vi "Generate Fully Qualified Channel Names.vi"() -> (1 "Rx channels":string[](array[string]), 2 "trigger channels":string[](array[string]), 3 "Tx channels":string[](array[string]), 4 "channel index":dbl[](array[numeric]))   [LabVIEW 2020, in "Single Core Acyclic Loopback.lvclass"]
uses:
  Single Core Acyclic Loopback.lvclass
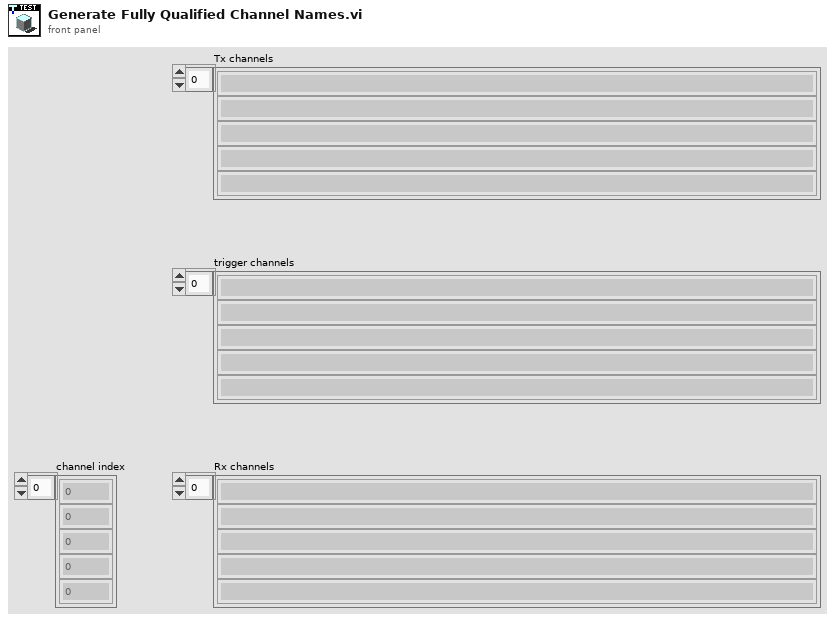
[diagram p1: front panel]
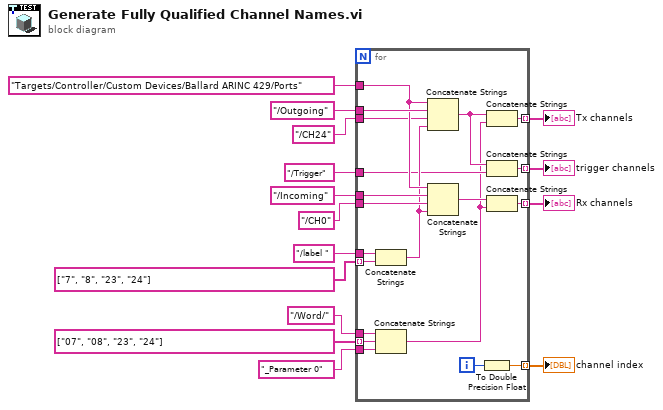
[diagram p0: block diagram]
diagram:
  n1 = for {
    tunnel: [w35] -> w14 mode=indexing
    tunnel: "Targets/Controller/Custom Devices/Ballard ARINC 429/Ports" ("Channel") -> [w27]
    tunnel: string[] ["07", "08", "23", "24"] -> [w33] mode=indexing
    tunnel: "_Parameter 0" ("format string") -> [w32]
    tunnel: "/label " ("format string") -> [w31]
    tunnel: string[] ["7", "8", "23", "24"] -> [w30] mode=indexing
    tunnel: "/Word/" ("input 1") -> [w29]
    tunnel: "/Outgoing" ("format string") -> [w28]
    tunnel: "/Incoming" ("format string") -> [w26]
    tunnel: "/CH0" ("format string") -> [w25]
    tunnel: "/CH24" ("format string") -> [w24]
    tunnel: "/Trigger" ("input 1") -> [w22]
    tunnel: [w21] -> w3 mode=indexing
    tunnel: [w17] -> w2 mode=indexing
    tunnel: [w16] -> w1 mode=indexing
    i -> [w34]
    n2 = Concatenate Strings(w31, w30) -> (w23:string)
    n3 = Concatenate Strings(w29, w33, w32) -> (w18:string)
    n4 = Concatenate Strings(w27, w28, w24, w23) -> (w19:string)
    n5 = Concatenate Strings(w27, w26, w25, w23) -> (w20:string)
    n6 = To Double Precision Float(number=w34) -> (double precision float=w35:dbl)
    n7 = Concatenate Strings(w19, w18) -> (w16:string)
    n8 = Concatenate Strings(w19, w22) -> (w21:string)
    n9 = Concatenate Strings(w20, w18) -> (w17:string)
  }
  "trigger channels" <- w3
  "Rx channels" <- w2
  "Tx channels" <- w1
  "channel index" <- w14
